vi "Setting SMU Range.vi"(1 "SMU - Sweeping":T2={"Start / Offset"=0.0, "Stop / Ratio"=1.0, "Step (linear only)"=0.01, "Compliance"=0.1, "Power Compliance"=0.0, "Mode"=0, "Function"=0, "Sweep Mode"=FALSE} caption="SMU" {"Function" items=["Disabled", "Var 1", "Var 2", "Var 1'", "Constant"]; "Mode" items=["V", "I", "V pulse", "I  pulse", "Common"]; "Power Compliance" format="%^.2e"; "Compliance" format="%^.2e"; "Step (linear only)" format="%^.4e"; "Stop / Ratio" format="%^.4e"; "Start / Offset" format="%^.4e"}, 2 "Range":u16(ring) items=["auto", "fixed", "limited"], 3 "unit (VMU1:0)":u16) -> (0 "output cluster":T1)   [LabVIEW 2014]
panel:
  # "LICENSED MATERIALS – PROPERTY OF IBM\nCopyright IBM Corp. 2016,\nALL RIGHTS RESERVED"
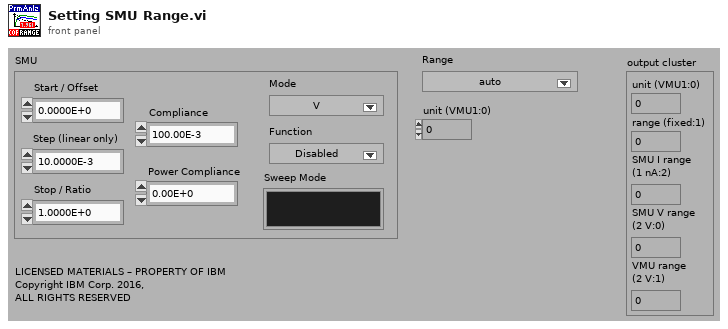
[diagram p1: front panel]
types:
  T1 = cluster{"unit (VMU1:0)":u16, "range (fixed:1)":u16, "SMU I range\n(1 nA:2)":u16, "SMU V range\n(2 V:0)":u16, "VMU range\n(2 V:1)":u16}
  T2 = cluster{"Start / Offset":dbl, "Stop / Ratio":dbl, "Step (linear only)":dbl, "Compliance":dbl, "Power Compliance":dbl, "Mode":u32, "Function":i32, "Sweep Mode":bool}
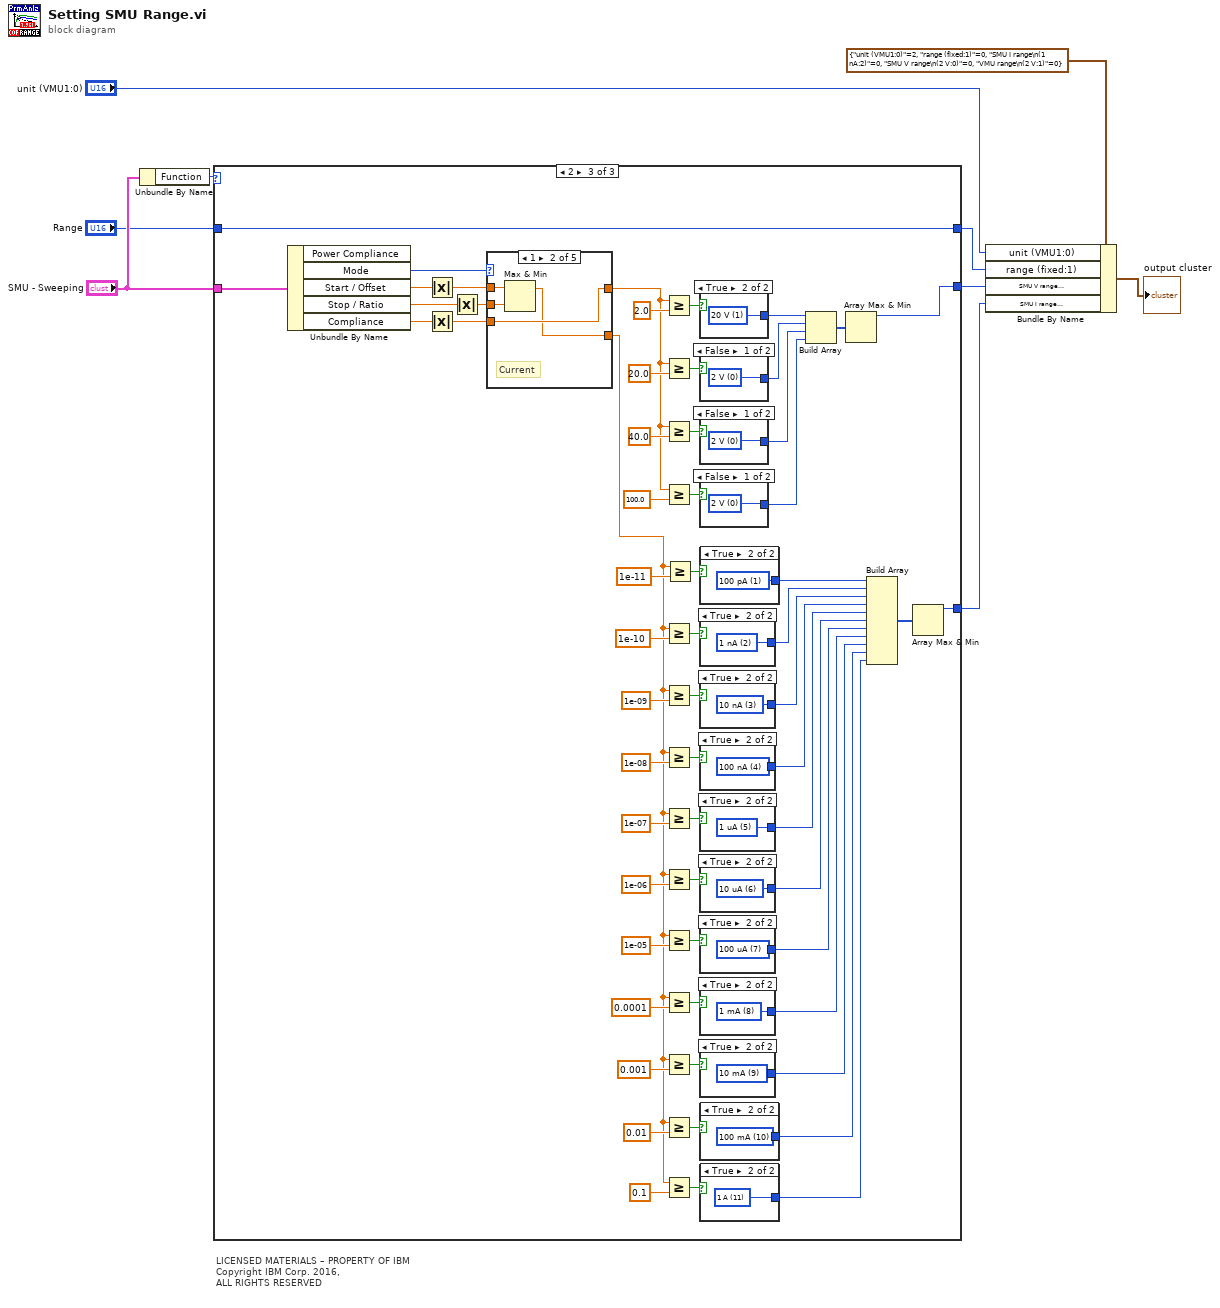
[diagram p0: block diagram]
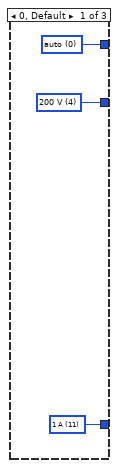
[diagram p2: hidden frame]
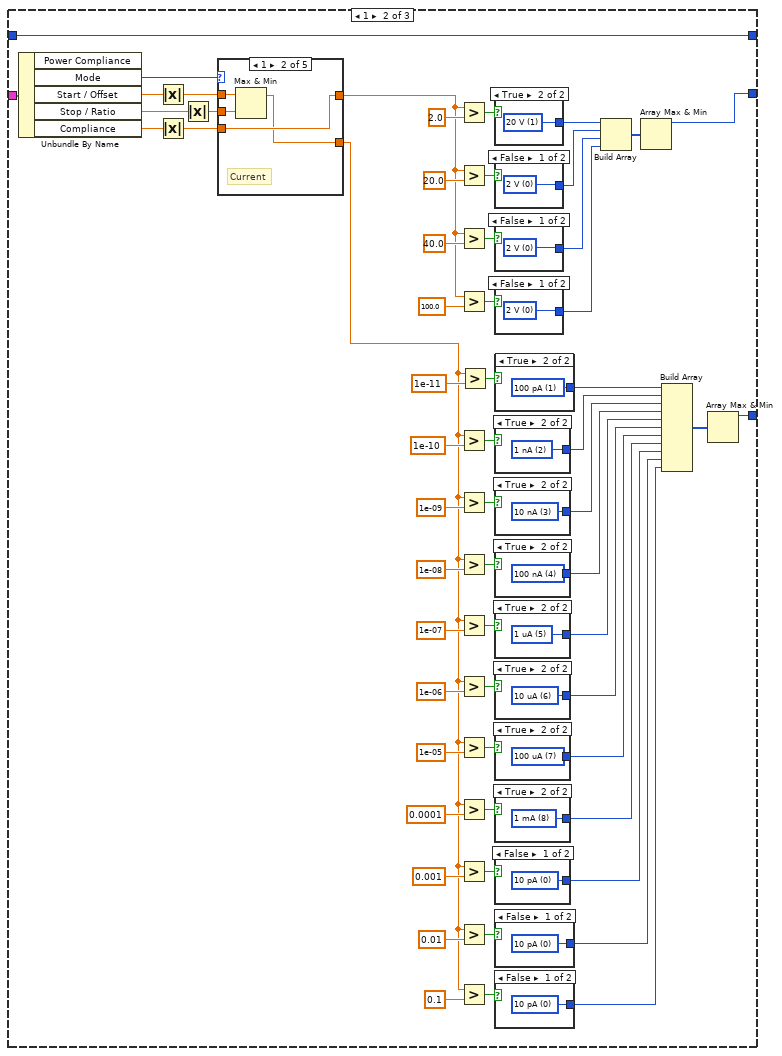
[diagram p3: hidden frame]
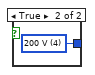
[diagram p4: hidden frame]
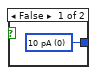
[diagram p5: hidden frame]
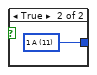
[diagram p6: hidden frame]
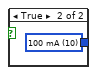
[diagram p7: hidden frame]
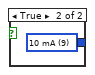
[diagram p8: hidden frame]
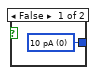
[diagram p9: hidden frame]
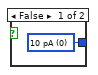
[diagram p10: hidden frame]
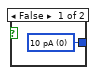
[diagram p11: hidden frame]
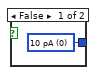
[diagram p12: hidden frame]
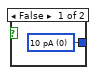
[diagram p13: hidden frame]
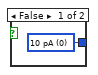
[diagram p14: hidden frame]
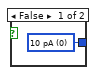
[diagram p15: hidden frame]
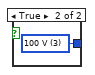
[diagram p16: hidden frame]
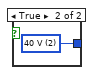
[diagram p17: hidden frame]
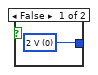
[diagram p18: hidden frame]
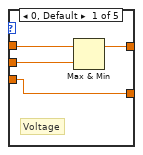
[diagram p19: hidden frame]
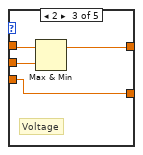
[diagram p20: hidden frame]
diagram:
  # "LICENSED MATERIALS – PROPERTY OF IBM\nCopyright IBM Corp. 2016,\nALL RIGHTS RESERVED"
  n1 = Unbundle By Name("SMU - Sweeping") -> ("Function"=w1:i32)
  n2 = case shown="2" w1 {
    tunnel: [w11 w55 w163] -> w7
    tunnel: [w10 w19 w127] -> w6
    tunnel: "SMU - Sweeping" -> [_ w14 w122]
    tunnel: "Range" -> [_ w13 w121]
    tunnel: [w12 w13 w121] -> w2
    frame 0, Default {
      w10 = u16 11 items=["10 pA", "100 pA", "1 nA", "10 nA", "100 nA", "1 uA", "10 uA", "100 uA", "1 mA", "10 mA", "100 mA", "1 A"] ("SMU I range\n(1 nA:2)")
      w11 = u16 4 items=["2 V", "20 V", "40 V", "100 V ", "200 V"] ("SMU V range\n(2 V:0)")
      w12 = u16 0 items=["auto", "fixed", "limited"] ("Range")
    }
    frame 1 {
      n3 = Unbundle By Name(w14) -> ("Mode"=w72:u32, "Start / Offset"=w71:dbl, "Stop / Ratio"=w70:dbl, "Compliance"=w69:dbl)  [unwired: 1 out]
      n4 = Absolute Value(x=w71) -> (abs(x)=w68:dbl)
      n5 = Absolute Value(x=w69) -> (abs(x)=w66:dbl)
      n6 = Absolute Value(x=w70) -> (abs(x)=w67:dbl)
      n7 = case shown="1" w72 {
        tunnel: w68 -> [w104 w109 w114 w118 _]
        tunnel: w67 -> [w103 w108 w113 w117 _]
        tunnel: w66 -> [w105 w110 w112 w115 _]
        tunnel: [w106 w110 w111 w115 0.0 ("Compliance")] -> w15
        tunnel: [w105 w107 w112 w116 0.0 ("Compliance")] -> w32
        frame 0, Default {
          # "Voltage"
          n8 = Max & Min(x=w104, y=w103) -> (max(x,y)=w106:dbl)  [unwired: 1 out]
        }
        frame 1 {
          # "Current"
          n9 = Max & Min(x=w109, y=w108) -> (max(x,y)=w107:dbl)  [unwired: 1 out]
        }
        frame 2 {
          # "Voltage"
          n10 = Max & Min(x=w114, y=w113) -> (max(x,y)=w111:dbl)  [unwired: 1 out]
        }
        frame 3 {
          # "Current"
          n11 = Max & Min(x=w118, y=w117) -> (max(x,y)=w116:dbl)  [unwired: 1 out]
        }
        frame 4 {
          # "Common"
        }
      }
      n12 = Greater?(x=w15, y=2.0 ("Compliance")) -> (0:w62:bool)
      n13 = Greater?(x=w15, y=20.0 ("Compliance")) -> (0:w61:bool)
      n14 = Greater?(x=w15, y=40.0 ("Compliance")) -> (0:w60:bool)
      n15 = Greater?(x=w15, y=100.0 ("Compliance")) -> (0:w18:bool)
      n16 = Greater?(x=w32, y=1e-10 ("Compliance")) -> (0:w44:bool)
      n17 = Greater?(x=w32, y=1e-09 ("Compliance")) -> (0:w43:bool)
      n18 = Greater?(x=w32, y=1e-08 ("Compliance")) -> (0:w42:bool)
      n19 = Greater?(x=w32, y=1e-07 ("Compliance")) -> (0:w41:bool)
      n20 = Greater?(x=w32, y=1e-06 ("Compliance")) -> (0:w40:bool)
      n21 = Greater?(x=w32, y=1e-05 ("Compliance")) -> (0:w39:bool)
      n22 = Greater?(x=w32, y=0.0001 ("Compliance")) -> (0:w38:bool)
      n23 = Greater?(x=w32, y=0.001 ("Compliance")) -> (0:w37:bool)
      n24 = Greater?(x=w32, y=0.01 ("Compliance")) -> (0:w36:bool)
      n25 = Greater?(x=w32, y=0.1 ("Compliance")) -> (0:w35:bool)
      n26 = Greater?(x=w32, y=1e-11 ("Compliance")) -> (0:w34:bool)
      n27 = case shown="True" w62 {
        tunnel: [w101 w102] -> w59
        frame False {
          w101 = u16 0 items=["2 V", "20 V", "40 V", "100 V ", "200 V"] ("SMU V range\n(2 V:0)")
        }
        frame True {
          w102 = u16 1 items=["2 V", "20 V", "40 V", "100 V ", "200 V"] ("SMU V range\n(2 V:0)")
        }
      }
      n28 = case shown="False" w61 {
        tunnel: [w99 w100] -> w58
        frame False {
          w99 = u16 0 items=["2 V", "20 V", "40 V", "100 V ", "200 V"] ("SMU V range\n(2 V:0)")
        }
        frame True {
          w100 = u16 2 items=["2 V", "20 V", "40 V", "100 V ", "200 V"] ("SMU V range\n(2 V:0)")
        }
      }
      n29 = case shown="False" w60 {
        tunnel: [w97 w98] -> w57
        frame False {
          w97 = u16 0 items=["2 V", "20 V", "40 V", "100 V ", "200 V"] ("SMU V range\n(2 V:0)")
        }
        frame True {
          w98 = u16 3 items=["2 V", "20 V", "40 V", "100 V ", "200 V"] ("SMU V range\n(2 V:0)")
        }
      }
      n30 = case shown="False" w18 {
        tunnel: [w73 w74] -> w16
        frame False {
          w73 = u16 0 items=["2 V", "20 V", "40 V", "100 V ", "200 V"] ("SMU V range\n(2 V:0)")
        }
        frame True {
          w74 = u16 4 items=["2 V", "20 V", "40 V", "100 V ", "200 V"] ("SMU V range\n(2 V:0)")
        }
      }
      n31 = case shown="True" w34 {
        tunnel: [w75 w76] -> w31
        frame False {
          w75 = u16 0 items=["10 pA", "100 pA", "1 nA", "10 nA", "100 nA", "1 uA", "10 uA", "100 uA", "1 mA", "10 mA", "100 mA", "1 A"] ("SMU I range\n(1 nA:2)")
        }
        frame True {
          w76 = u16 1 items=["10 pA", "100 pA", "1 nA", "10 nA", "100 nA", "1 uA", "10 uA", "100 uA", "1 mA", "10 mA", "100 mA", "1 A"] ("SMU I range\n(1 nA:2)")
        }
      }
      n32 = case shown="True" w44 {
        tunnel: [w95 w96] -> w30
        frame False {
          w95 = u16 0 items=["10 pA", "100 pA", "1 nA", "10 nA", "100 nA", "1 uA", "10 uA", "100 uA", "1 mA", "10 mA", "100 mA", "1 A"] ("SMU I range\n(1 nA:2)")
        }
        frame True {
          w96 = u16 2 items=["10 pA", "100 pA", "1 nA", "10 nA", "100 nA", "1 uA", "10 uA", "100 uA", "1 mA", "10 mA", "100 mA", "1 A"] ("SMU I range\n(1 nA:2)")
        }
      }
      n33 = case shown="True" w43 {
        tunnel: [w93 w94] -> w29
        frame False {
          w93 = u16 0 items=["10 pA", "100 pA", "1 nA", "10 nA", "100 nA", "1 uA", "10 uA", "100 uA", "1 mA", "10 mA", "100 mA", "1 A"] ("SMU I range\n(1 nA:2)")
        }
        frame True {
          w94 = u16 3 items=["10 pA", "100 pA", "1 nA", "10 nA", "100 nA", "1 uA", "10 uA", "100 uA", "1 mA", "10 mA", "100 mA", "1 A"] ("SMU I range\n(1 nA:2)")
        }
      }
      n34 = case shown="True" w42 {
        tunnel: [w91 w92] -> w28
        frame False {
          w91 = u16 0 items=["10 pA", "100 pA", "1 nA", "10 nA", "100 nA", "1 uA", "10 uA", "100 uA", "1 mA", "10 mA", "100 mA", "1 A"] ("SMU I range\n(1 nA:2)")
        }
        frame True {
          w92 = u16 4 items=["10 pA", "100 pA", "1 nA", "10 nA", "100 nA", "1 uA", "10 uA", "100 uA", "1 mA", "10 mA", "100 mA", "1 A"] ("SMU I range\n(1 nA:2)")
        }
      }
      n35 = case shown="True" w41 {
        tunnel: [w89 w90] -> w26
        frame False {
          w89 = u16 0 items=["10 pA", "100 pA", "1 nA", "10 nA", "100 nA", "1 uA", "10 uA", "100 uA", "1 mA", "10 mA", "100 mA", "1 A"] ("SMU I range\n(1 nA:2)")
        }
        frame True {
          w90 = u16 5 items=["10 pA", "100 pA", "1 nA", "10 nA", "100 nA", "1 uA", "10 uA", "100 uA", "1 mA", "10 mA", "100 mA", "1 A"] ("SMU I range\n(1 nA:2)")
        }
      }
      n36 = case shown="True" w40 {
        tunnel: [w87 w88] -> w25
        frame False {
          w87 = u16 0 items=["10 pA", "100 pA", "1 nA", "10 nA", "100 nA", "1 uA", "10 uA", "100 uA", "1 mA", "10 mA", "100 mA", "1 A"] ("SMU I range\n(1 nA:2)")
        }
        frame True {
          w88 = u16 6 items=["10 pA", "100 pA", "1 nA", "10 nA", "100 nA", "1 uA", "10 uA", "100 uA", "1 mA", "10 mA", "100 mA", "1 A"] ("SMU I range\n(1 nA:2)")
        }
      }
      n37 = case shown="True" w39 {
        tunnel: [w85 w86] -> w24
        frame False {
          w85 = u16 0 items=["10 pA", "100 pA", "1 nA", "10 nA", "100 nA", "1 uA", "10 uA", "100 uA", "1 mA", "10 mA", "100 mA", "1 A"] ("SMU I range\n(1 nA:2)")
        }
        frame True {
          w86 = u16 7 items=["10 pA", "100 pA", "1 nA", "10 nA", "100 nA", "1 uA", "10 uA", "100 uA", "1 mA", "10 mA", "100 mA", "1 A"] ("SMU I range\n(1 nA:2)")
        }
      }
      n38 = case shown="True" w38 {
        tunnel: [w83 w84] -> w23
        frame False {
          w83 = u16 0 items=["10 pA", "100 pA", "1 nA", "10 nA", "100 nA", "1 uA", "10 uA", "100 uA", "1 mA", "10 mA", "100 mA", "1 A"] ("SMU I range\n(1 nA:2)")
        }
        frame True {
          w84 = u16 8 items=["10 pA", "100 pA", "1 nA", "10 nA", "100 nA", "1 uA", "10 uA", "100 uA", "1 mA", "10 mA", "100 mA", "1 A"] ("SMU I range\n(1 nA:2)")
        }
      }
      n39 = case shown="False" w37 {
        tunnel: [w81 w82] -> w22
        frame False {
          w81 = u16 0 items=["10 pA", "100 pA", "1 nA", "10 nA", "100 nA", "1 uA", "10 uA", "100 uA", "1 mA", "10 mA", "100 mA", "1 A"] ("SMU I range\n(1 nA:2)")
        }
        frame True {
          w82 = u16 9 items=["10 pA", "100 pA", "1 nA", "10 nA", "100 nA", "1 uA", "10 uA", "100 uA", "1 mA", "10 mA", "100 mA", "1 A"] ("SMU I range\n(1 nA:2)")
        }
      }
      n40 = case shown="False" w36 {
        tunnel: [w79 w80] -> w21
        frame False {
          w79 = u16 0 items=["10 pA", "100 pA", "1 nA", "10 nA", "100 nA", "1 uA", "10 uA", "100 uA", "1 mA", "10 mA", "100 mA", "1 A"] ("SMU I range\n(1 nA:2)")
        }
        frame True {
          w80 = u16 10 items=["10 pA", "100 pA", "1 nA", "10 nA", "100 nA", "1 uA", "10 uA", "100 uA", "1 mA", "10 mA", "100 mA", "1 A"] ("SMU I range\n(1 nA:2)")
        }
      }
      n41 = case shown="False" w35 {
        tunnel: [w77 w78] -> w27
        frame False {
          w77 = u16 0 items=["10 pA", "100 pA", "1 nA", "10 nA", "100 nA", "1 uA", "10 uA", "100 uA", "1 mA", "10 mA", "100 mA", "1 A"] ("SMU I range\n(1 nA:2)")
        }
        frame True {
          w78 = u16 11 items=["10 pA", "100 pA", "1 nA", "10 nA", "100 nA", "1 uA", "10 uA", "100 uA", "1 mA", "10 mA", "100 mA", "1 A"] ("SMU I range\n(1 nA:2)")
        }
      }
      n42 = Build Array(w59, w58, w57, w16) -> (w56:u16[])
      n43 = Array Max & Min(array=w56) -> (max value=w55:u16)  [unwired: 3 out]
      n44 = Build Array(w31, w30, w29, w28, w26, w25, w24, w23, w22, w21, w27) -> (w20:u16[])
      n45 = Array Max & Min(array=w20) -> (max value=w19:u16)  [unwired: 3 out]
    }
    frame 2 {
      n46 = Unbundle By Name(w122) -> ("Mode"=w180:u32, "Start / Offset"=w179:dbl, "Stop / Ratio"=w178:dbl, "Compliance"=w177:dbl)  [unwired: 1 out]
      n47 = Absolute Value(x=w179) -> (abs(x)=w176:dbl)
      n48 = Absolute Value(x=w177) -> (abs(x)=w174:dbl)
      n49 = Absolute Value(x=w178) -> (abs(x)=w175:dbl)
      n50 = case shown="1" w180 {
        tunnel: w176 -> [w212 w217 w222 w226 _]
        tunnel: w175 -> [w211 w216 w221 w225 _]
        tunnel: w174 -> [w213 w218 w220 w223 _]
        tunnel: [w214 w218 w219 w223 0.0 ("Compliance")] -> w123
        tunnel: [w213 w215 w220 w224 0.0 ("Compliance")] -> w140
        frame 0, Default {
          # "Voltage"
          n51 = Max & Min(x=w212, y=w211) -> (max(x,y)=w214:dbl)  [unwired: 1 out]
        }
        frame 1 {
          # "Current"
          n52 = Max & Min(x=w217, y=w216) -> (max(x,y)=w215:dbl)  [unwired: 1 out]
        }
        frame 2 {
          # "Voltage"
          n53 = Max & Min(x=w222, y=w221) -> (max(x,y)=w219:dbl)  [unwired: 1 out]
        }
        frame 3 {
          # "Current"
          n54 = Max & Min(x=w226, y=w225) -> (max(x,y)=w224:dbl)  [unwired: 1 out]
        }
        frame 4 {
          # "Common"
        }
      }
      n55 = Greater Or Equal?(x=w123, y=2.0 ("Compliance")) -> (x >= y?=w170:bool)
      n56 = Greater Or Equal?(x=w123, y=20.0 ("Compliance")) -> (x >= y?=w169:bool)
      n57 = Greater Or Equal?(x=w123, y=40.0 ("Compliance")) -> (x >= y?=w168:bool)
      n58 = Greater Or Equal?(x=w123, y=100.0 ("Compliance")) -> (x >= y?=w126:bool)
      n59 = Greater Or Equal?(x=w140, y=1e-10 ("Compliance")) -> (x >= y?=w152:bool)
      n60 = Greater Or Equal?(x=w140, y=1e-09 ("Compliance")) -> (x >= y?=w151:bool)
      n61 = Greater Or Equal?(x=w140, y=1e-08 ("Compliance")) -> (x >= y?=w150:bool)
      n62 = Greater Or Equal?(x=w140, y=1e-07 ("Compliance")) -> (x >= y?=w149:bool)
      n63 = Greater Or Equal?(x=w140, y=1e-06 ("Compliance")) -> (x >= y?=w148:bool)
      n64 = Greater Or Equal?(x=w140, y=1e-05 ("Compliance")) -> (x >= y?=w147:bool)
      n65 = Greater Or Equal?(x=w140, y=0.0001 ("Compliance")) -> (x >= y?=w146:bool)
      n66 = Greater Or Equal?(x=w140, y=0.001 ("Compliance")) -> (x >= y?=w145:bool)
      n67 = Greater Or Equal?(x=w140, y=0.01 ("Compliance")) -> (x >= y?=w144:bool)
      n68 = Greater Or Equal?(x=w140, y=0.1 ("Compliance")) -> (x >= y?=w143:bool)
      n69 = Greater Or Equal?(x=w140, y=1e-11 ("Compliance")) -> (x >= y?=w142:bool)
      n70 = case shown="True" w170 {
        tunnel: [w209 w210] -> w167
        frame False {
          w209 = u16 0 items=["2 V", "20 V", "40 V", "100 V ", "200 V"] ("SMU V range\n(2 V:0)")
        }
        frame True {
          w210 = u16 1 items=["2 V", "20 V", "40 V", "100 V ", "200 V"] ("SMU V range\n(2 V:0)")
        }
      }
      n71 = case shown="False" w169 {
        tunnel: [w207 w208] -> w166
        frame False {
          w207 = u16 0 items=["2 V", "20 V", "40 V", "100 V ", "200 V"] ("SMU V range\n(2 V:0)")
        }
        frame True {
          w208 = u16 2 items=["2 V", "20 V", "40 V", "100 V ", "200 V"] ("SMU V range\n(2 V:0)")
        }
      }
      n72 = case shown="False" w168 {
        tunnel: [w205 w206] -> w165
        frame False {
          w205 = u16 0 items=["2 V", "20 V", "40 V", "100 V ", "200 V"] ("SMU V range\n(2 V:0)")
        }
        frame True {
          w206 = u16 3 items=["2 V", "20 V", "40 V", "100 V ", "200 V"] ("SMU V range\n(2 V:0)")
        }
      }
      n73 = case shown="False" w126 {
        tunnel: [w181 w182] -> w124
        frame False {
          w181 = u16 0 items=["2 V", "20 V", "40 V", "100 V ", "200 V"] ("SMU V range\n(2 V:0)")
        }
        frame True {
          w182 = u16 4 items=["2 V", "20 V", "40 V", "100 V ", "200 V"] ("SMU V range\n(2 V:0)")
        }
      }
      n74 = case shown="True" w142 {
        tunnel: [w183 w184] -> w139
        frame False {
          w183 = u16 0 items=["10 pA", "100 pA", "1 nA", "10 nA", "100 nA", "1 uA", "10 uA", "100 uA", "1 mA", "10 mA", "100 mA", "1 A"] ("SMU I range\n(1 nA:2)")
        }
        frame True {
          w184 = u16 1 items=["10 pA", "100 pA", "1 nA", "10 nA", "100 nA", "1 uA", "10 uA", "100 uA", "1 mA", "10 mA", "100 mA", "1 A"] ("SMU I range\n(1 nA:2)")
        }
      }
      n75 = case shown="True" w152 {
        tunnel: [w203 w204] -> w138
        frame False {
          w203 = u16 0 items=["10 pA", "100 pA", "1 nA", "10 nA", "100 nA", "1 uA", "10 uA", "100 uA", "1 mA", "10 mA", "100 mA", "1 A"] ("SMU I range\n(1 nA:2)")
        }
        frame True {
          w204 = u16 2 items=["10 pA", "100 pA", "1 nA", "10 nA", "100 nA", "1 uA", "10 uA", "100 uA", "1 mA", "10 mA", "100 mA", "1 A"] ("SMU I range\n(1 nA:2)")
        }
      }
      n76 = case shown="True" w151 {
        tunnel: [w201 w202] -> w137
        frame False {
          w201 = u16 0 items=["10 pA", "100 pA", "1 nA", "10 nA", "100 nA", "1 uA", "10 uA", "100 uA", "1 mA", "10 mA", "100 mA", "1 A"] ("SMU I range\n(1 nA:2)")
        }
        frame True {
          w202 = u16 3 items=["10 pA", "100 pA", "1 nA", "10 nA", "100 nA", "1 uA", "10 uA", "100 uA", "1 mA", "10 mA", "100 mA", "1 A"] ("SMU I range\n(1 nA:2)")
        }
      }
      n77 = case shown="True" w150 {
        tunnel: [w199 w200] -> w136
        frame False {
          w199 = u16 0 items=["10 pA", "100 pA", "1 nA", "10 nA", "100 nA", "1 uA", "10 uA", "100 uA", "1 mA", "10 mA", "100 mA", "1 A"] ("SMU I range\n(1 nA:2)")
        }
        frame True {
          w200 = u16 4 items=["10 pA", "100 pA", "1 nA", "10 nA", "100 nA", "1 uA", "10 uA", "100 uA", "1 mA", "10 mA", "100 mA", "1 A"] ("SMU I range\n(1 nA:2)")
        }
      }
      n78 = case shown="True" w149 {
        tunnel: [w197 w198] -> w134
        frame False {
          w197 = u16 0 items=["10 pA", "100 pA", "1 nA", "10 nA", "100 nA", "1 uA", "10 uA", "100 uA", "1 mA", "10 mA", "100 mA", "1 A"] ("SMU I range\n(1 nA:2)")
        }
        frame True {
          w198 = u16 5 items=["10 pA", "100 pA", "1 nA", "10 nA", "100 nA", "1 uA", "10 uA", "100 uA", "1 mA", "10 mA", "100 mA", "1 A"] ("SMU I range\n(1 nA:2)")
        }
      }
      n79 = case shown="True" w148 {
        tunnel: [w195 w196] -> w133
        frame False {
          w195 = u16 0 items=["10 pA", "100 pA", "1 nA", "10 nA", "100 nA", "1 uA", "10 uA", "100 uA", "1 mA", "10 mA", "100 mA", "1 A"] ("SMU I range\n(1 nA:2)")
        }
        frame True {
          w196 = u16 6 items=["10 pA", "100 pA", "1 nA", "10 nA", "100 nA", "1 uA", "10 uA", "100 uA", "1 mA", "10 mA", "100 mA", "1 A"] ("SMU I range\n(1 nA:2)")
        }
      }
      n80 = case shown="True" w147 {
        tunnel: [w193 w194] -> w132
        frame False {
          w193 = u16 0 items=["10 pA", "100 pA", "1 nA", "10 nA", "100 nA", "1 uA", "10 uA", "100 uA", "1 mA", "10 mA", "100 mA", "1 A"] ("SMU I range\n(1 nA:2)")
        }
        frame True {
          w194 = u16 7 items=["10 pA", "100 pA", "1 nA", "10 nA", "100 nA", "1 uA", "10 uA", "100 uA", "1 mA", "10 mA", "100 mA", "1 A"] ("SMU I range\n(1 nA:2)")
        }
      }
      n81 = case shown="True" w146 {
        tunnel: [w191 w192] -> w131
        frame False {
          w191 = u16 0 items=["10 pA", "100 pA", "1 nA", "10 nA", "100 nA", "1 uA", "10 uA", "100 uA", "1 mA", "10 mA", "100 mA", "1 A"] ("SMU I range\n(1 nA:2)")
        }
        frame True {
          w192 = u16 8 items=["10 pA", "100 pA", "1 nA", "10 nA", "100 nA", "1 uA", "10 uA", "100 uA", "1 mA", "10 mA", "100 mA", "1 A"] ("SMU I range\n(1 nA:2)")
        }
      }
      n82 = case shown="True" w145 {
        tunnel: [w189 w190] -> w130
        frame False {
          w189 = u16 0 items=["10 pA", "100 pA", "1 nA", "10 nA", "100 nA", "1 uA", "10 uA", "100 uA", "1 mA", "10 mA", "100 mA", "1 A"] ("SMU I range\n(1 nA:2)")
        }
        frame True {
          w190 = u16 9 items=["10 pA", "100 pA", "1 nA", "10 nA", "100 nA", "1 uA", "10 uA", "100 uA", "1 mA", "10 mA", "100 mA", "1 A"] ("SMU I range\n(1 nA:2)")
        }
      }
      n83 = case shown="True" w144 {
        tunnel: [w187 w188] -> w129
        frame False {
          w187 = u16 0 items=["10 pA", "100 pA", "1 nA", "10 nA", "100 nA", "1 uA", "10 uA", "100 uA", "1 mA", "10 mA", "100 mA", "1 A"] ("SMU I range\n(1 nA:2)")
        }
        frame True {
          w188 = u16 10 items=["10 pA", "100 pA", "1 nA", "10 nA", "100 nA", "1 uA", "10 uA", "100 uA", "1 mA", "10 mA", "100 mA", "1 A"] ("SMU I range\n(1 nA:2)")
        }
      }
      n84 = case shown="True" w143 {
        tunnel: [w185 w186] -> w135
        frame False {
          w185 = u16 0 items=["10 pA", "100 pA", "1 nA", "10 nA", "100 nA", "1 uA", "10 uA", "100 uA", "1 mA", "10 mA", "100 mA", "1 A"] ("SMU I range\n(1 nA:2)")
        }
        frame True {
          w186 = u16 11 items=["10 pA", "100 pA", "1 nA", "10 nA", "100 nA", "1 uA", "10 uA", "100 uA", "1 mA", "10 mA", "100 mA", "1 A"] ("SMU I range\n(1 nA:2)")
        }
      }
      n85 = Build Array(w167, w166, w165, w124) -> (w164:u16[])
      n86 = Array Max & Min(array=w164) -> (max value=w163:u16)  [unwired: 3 out]
      n87 = Build Array(w139, w138, w137, w136, w134, w133, w132, w131, w130, w129, w135) -> (w128:u16[])
      n88 = Array Max & Min(array=w128) -> (max value=w127:u16)  [unwired: 3 out]
    }
  }
  n89 = Bundle By Name(cluster=T1 {"unit (VMU1:0)"=2, "range (fixed:1)"=0, "SMU I range\n(1 nA:2)"=0, "SMU V range\n(2 V:0)"=0, "VMU range\n(2 V:1)"=0}, "unit (VMU1:0)"="unit (VMU1:0)", "range (fixed:1)"=w2, "SMU V range\n(2 V:0)"=w7, "SMU I range\n(1 nA:2)"=w6) -> (→"output cluster":T1)
